vi "TakeSingleImage.vi"(0 "Image":T1, 1 "TLCamera reference in":refnum<k24>, 2 "ExposureTime_us":u32, 3 "Error In":errorcluster) -> (7 "Image Out":T1, 8 "TLCamera reference out":refnum<k24>, 10 "Error Out":errorcluster)   [LabVIEW 2019]
uses:
  <vilib>/vision/Image Controls.llb/IMAQ Image.ctl
  C:/Users/jleeman/git_repos/CAxis_Machine/C-Axis LabView Controller/Library_X64/Thorlabs.TSI.TLCameraInterfaces.dll
  Library_X64/Thorlabs.TSI.TLCameraInterfaces.dll
panel:
  out "Array":u16[][](array[numeric])
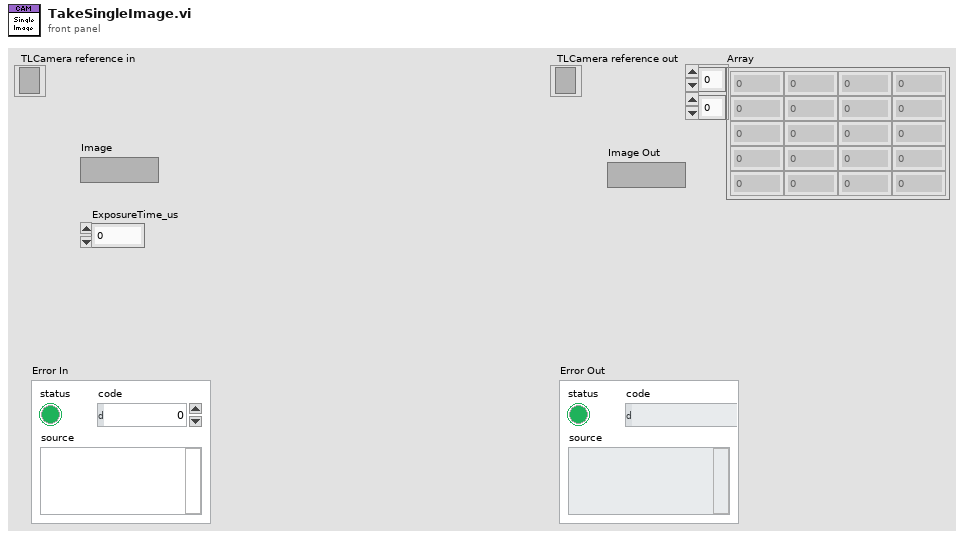
[diagram p1: front panel]
types:
  T1 = typedef "IMAQ Image.ctl" = refnum<image>
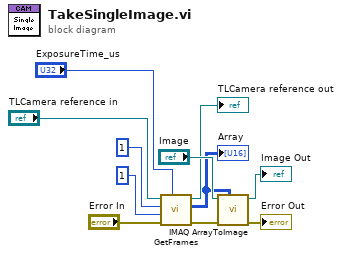
[diagram p0: block diagram]
diagram:
  n1 = call "GetFrames.vi"("ExposureTime_us"="ExposureTime_us", "Error In"="Error In", "FramesPerTrigger"=u32 1, "Gain"=u32 1, "TLCamera reference in"="TLCamera reference in") -> ("Error Out"=w6:errorcluster, "Array"=w7:u16[][], "TLCamera reference out"=→"TLCamera reference out":refnum<k24>)  [unwired: 4 in]
  "Array" <- w7
  n2 = call "IMAQ ArrayToImage"("Image Pixels (U16)"=w7, "error in (no error)"=w6, "Image"="Image") -> ("error out"=→"Error Out":errorcluster, "Image Out"=→"Image Out":T1)  [unwired: 7 in]
